vi "myRIO_BRig_Host_test_dataGeneration_correctData.vi"(10 "input_nTrial_perBlock":u16, 11 "input_nTrial_total":u16) -> (3 "output_correctData":u16[][](array[numeric]))   [LabVIEW 2014]
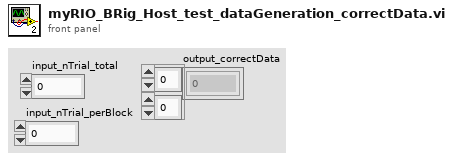
[diagram p1: front panel]
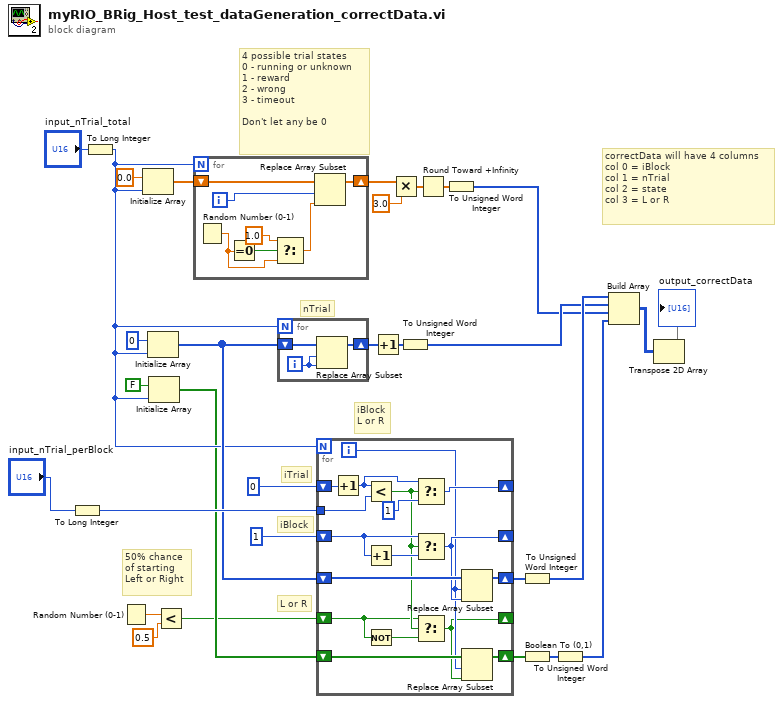
[diagram p0: block diagram]
diagram:
  # "50% chance\nof starting\nLeft or Right"
  # "L or R"
  # "iBlock"
  # "iTrial"
  # "iBlock\nL or R"
  # "nTrial"
  # "correctData will have 4 columns\ncol 0 = iBlock\ncol 1 = nTrial\ncol 2 = state\ncol 3 = L or R"
  # "4 possible trial states\n0 - running or unknown\n1 - reward\n2 - wrong\n3 - timeout\n\nDon't let any be 0"
  n1 = To Long Integer(number="input_nTrial_perBlock") -> (32bit integer=w20:i32)
  n2 = To Long Integer(number="input_nTrial_total") -> (32bit integer=w14:i32)
  n3 = Random Number (0-1)() -> (number: 0 to 1=w12:dbl)
  n4 = Initialize Array(0.0 ("element"), w14) -> (w24:dbl[])
  n5 = Initialize Array(0 ("element"), w14) -> (w16:i32[])
  n6 = Initialize Array(FALSE, w14) -> (w13:bool[])
  n7 = Less?(x=w12, y=0.5) -> (x < y?=w10:bool)
  n8 = for {
    N: w14 -> [_]
    shift-right: [w34] -> w28
    shift-left: w24 -> [w35]
    i -> [w32]
    n9 = Random Number (0-1)() -> (number: 0 to 1=w36:dbl)
    n10 = Equal To 0?(x=w36) -> (x = 0?=w37:bool)
    n11 = Select(t=1.0, s=w37, f=w36) -> (s? t:f=w31:dbl)
    n12 = Replace Array Subset(array=w35, new element=w31, index=w32) -> (w34:dbl[])
  }
  n13 = for {
    N: w14 -> [_]
    shift-right: [w39] -> w23
    shift-left: w16 -> [w40]
    i -> [w38]
    n14 = Replace Array Subset(array=w40, new element=w38, index=w38) -> (w39:i32[])
  }
  n15 = for {
    N: w14 -> [_]
    shift-right: [w53] -> _
    shift-left: 0 -> [w57]
    tunnel: w20 -> [w56]
    shift-right: [w48] -> _
    shift-left: 1 -> [w51]
    shift-right: [w49] -> w9
    shift-left: w16 -> [w50]
    shift-right: [w41] -> _
    shift-left: w10 -> [w45]
    shift-right: [w43] -> w8
    shift-left: w13 -> [w44]
    i -> [w42]
    n16 = Increment(x=w57) -> (x+1=w55:i32)
    n17 = Less?(x=w55, y=w56) -> (x < y?=w47:bool)
    n18 = Increment(x=w51) -> (x+1=w52:i32)
    n19 = Not(x=w45) -> (.not. x?=w46:bool)
    n20 = Select(t=w55, s=w47, f=1) -> (s? t:f=w53:i32)
    n21 = Select(t=w51, s=w47, f=w52) -> (s? t:f=w48:i32)
    n22 = Select(t=w45, s=w47, f=w46) -> (s? t:f=w41:bool)
    n23 = Replace Array Subset(array=w50, new element=w48, index=w42) -> (w49:i32[])
    n24 = Replace Array Subset(array=w44, new element=w41, index=w42) -> (w43:bool[])
  }
  n25 = Increment(x=w23) -> (x+1=w22:i32[])
  n26 = Multiply(x=w28, y=3.0 ("t")) -> (x*y=w26:dbl[])
  n27 = To Unsigned Word Integer(number=w22) -> (unsigned 16bit integer=w2:u16[])
  n28 = Round Toward +Infinity(x=w26) -> (ceil(x): smallest int >= x=w25:dbl[])
  n29 = To Unsigned Word Integer(number=w25) -> (unsigned 16bit integer=w1:u16[])
  n30 = To Unsigned Word Integer(number=w9) -> (unsigned 16bit integer=w5:u16[])
  n31 = Boolean To (0,1)(Boolean=w8) -> (0, 1=w7:i16[])
  n32 = To Unsigned Word Integer(number=w7) -> (unsigned 16bit integer=w6:u16[])
  n33 = Build Array(w5, w2, w1, w6) -> (w4:u16[][])
  n34 = Transpose 2D Array(2D array=w4) -> (transposed array=→"output_correctData":u16[][])
